vi "Auton - Center Gear.vi"(11 "Auton States":T1=enum."Reset Encoders") -> ()   [LabVIEW 2016]
uses:
  Auton - Center Gear States.ctl
  Robot Values.vi
  Vision Global.vi
panel:
  in  "Turn Setpoint to Mount Peg":dbl=9.0 format="%#_13g"
  in  "Mount Peg Distance SP":dbl=8.0
  out "Current State":T1
  in  "Back Away SP":dbl=-24.0
  in  "Drive Forward SP":dbl=60.0
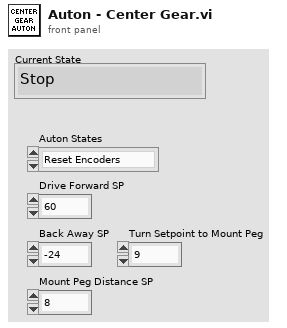
[diagram p1: front panel]
types:
  T1 = typedef "Auton - Center Gear States.ctl" = enum16{"Stop", "Wait For Target", "Reset Encoders", "Drive Forward", "Turn  To Mount Peg", "Reset Encoders Again", "Mount Peg", "Eject Gear", "Back Away"}
  T2 = typedef "Robot Values.ctl" = cluster{"Robot Drive":cluster{"Left Motor Power":dbl, "Right Motor Power":dbl, "Left Encoder Value":dbl, "Right Encoder Value":dbl, "High Gear?":bool, "PTO?":bool}, "Sensors":cluster{"Gyro Angle":u16, "Recalibrate Gyro":bool, "Reset Gyro":bool, "Ultrasonic":dbl}, "Shooter":cluster{"Prep Wheels":bool, "Shoot":bool, "Left Shooter Wheel Speed":dbl, "Wheels Moving":bool, "Shooter Prepped":bool, "Shooter RPS SP":dbl, "Shooting?":bool, "Left Shooter Wheel Power":dbl, "Right Shooter Wheel Power":dbl, "Acquisition Conveyor Power":dbl, "Hopper Beater Bar Power":dbl, "Filtered Left Shooter Speed":dbl, "Acquisition Motor Power":dbl, "Joystick Add":dbl, "D-Pad Add":dbl, "Shooter Use PID?":bool}, "Robot States":cluster{"Drive mode":string, "Alliance":T3, "Position":T4}, "Gear":cluster{"Ejection Active":bool}}
  T3 = typedef "WPI_DriverStationAllianceInfo.ctl" = enum16{"Red", "Blue", "Invalid"}
  T4 = typedef "WPI_DriverStationPositionInfo.ctl" = enum16{"1", "2", "3"}
  T5 = cluster{"Distance (ft)":dbl, "Score":dbl, "Normalized":cluster{"Center":cluster{dbl, dbl}, "Rectangle":cluster{"Numeric":dbl, "Numeric 2":dbl, "Numeric 3":dbl, "Numeric 5":dbl}}, "Pixels":cluster{"Center":cluster{dbl, dbl}, "Rectangle":cluster{"Numeric":dbl, "Numeric 2":dbl, "Numeric 3":dbl, "Numeric 5":dbl}}}
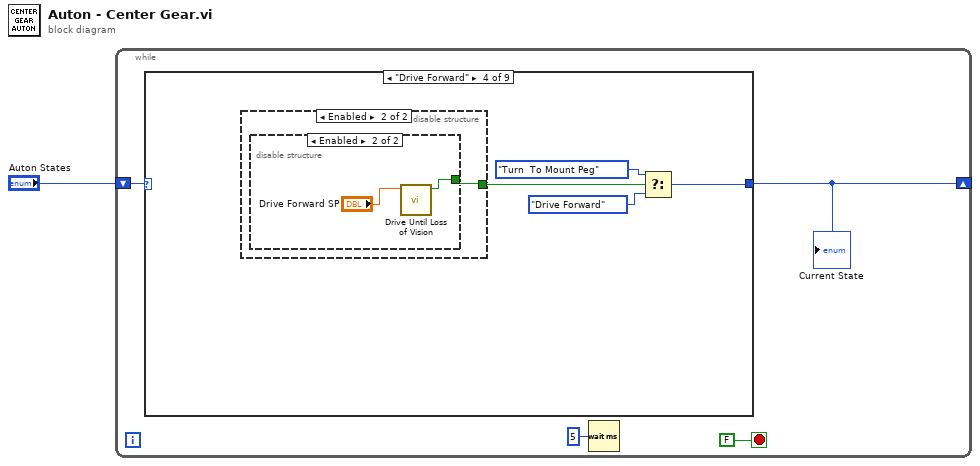
[diagram p0: block diagram]
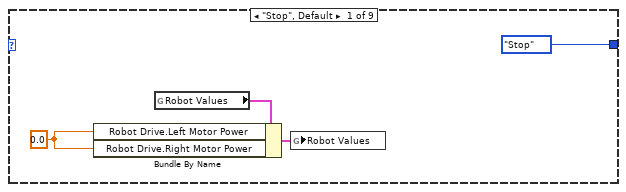
[diagram p2: hidden frame]
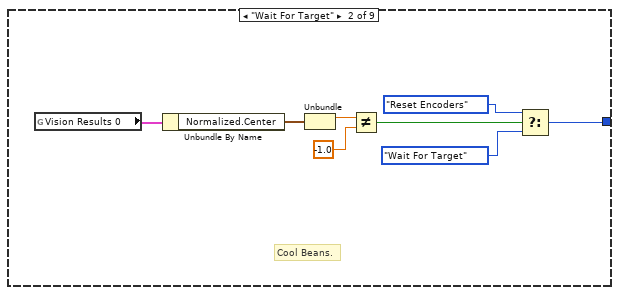
[diagram p3: hidden frame]
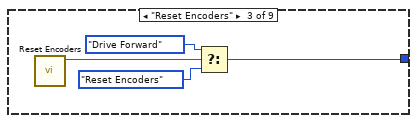
[diagram p4: hidden frame]
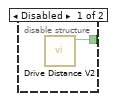
[diagram p5: hidden frame]
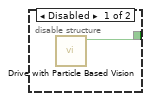
[diagram p6: hidden frame]
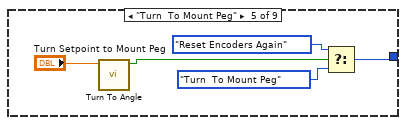
[diagram p7: hidden frame]
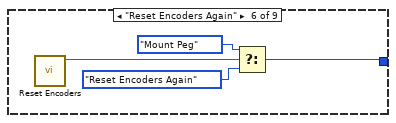
[diagram p8: hidden frame]
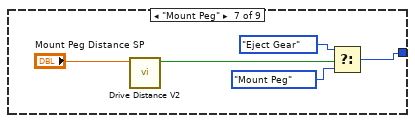
[diagram p9: hidden frame]
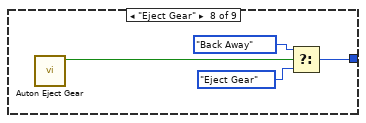
[diagram p10: hidden frame]
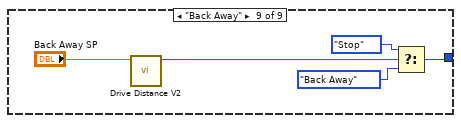
[diagram p11: hidden frame]
diagram:
  n1 = while {
    shift-right: [w4] -> _
    shift-left: "Auton States" -> [w5]
    stop <- FALSE stop-if-true
    n2 = case shown="\"Drive Forward\"" w5 {
      tunnel: [Auton_-_Center_Gear_States."Stop" ("Auton States 2") w17 w19 w23 w34 w37 w42 w47 w52] -> w4
      frame "Stop", Default {
        w6 = 0.0
        n3 = global read "Robot Values.vi" "Robot Values"() -> (w7:T2)
        n4 = Bundle By Name(cluster=w7, "Robot Drive.Left Motor Power"=w6, "Robot Drive.Right Motor Power"=w6) -> (w8:T2)
        n5 = global write "Robot Values.vi" "Robot Values"(w8) -> ()
      }
      frame "Wait For Target" {
        # "Cool Beans."
        n6 = global read "Vision Global.vi" "Vision Results 0"() -> (w14:T5)
        n7 = Unbundle By Name(w14) -> ("Normalized.Center"=w13:cluster{dbl, dbl})
        n8 = Unbundle(w13) -> (w12:dbl)  [unwired: 1 out]
        n9 = Not Equal?(x=w12, y=-1.0) -> (x != y?=w10:bool)
        n10 = Select(t=Auton_-_Center_Gear_States."Reset Encoders" ("Auton States 2"), s=w10, f=Auton_-_Center_Gear_States."Wait For Target") -> (s? t:f=w17:T1)
      }
      frame "Reset Encoders" {
        n11 = call "Reset Encoders.vi"() -> ("Done?"=w18:bool)  [unwired: 11 in]
        n12 = Select(t=Auton_-_Center_Gear_States."Drive Forward" ("Auton States 2"), s=w18, f=Auton_-_Center_Gear_States."Reset Encoders" ("Auton States 2")) -> (s? t:f=w19:T1)
      }
      frame "Drive Forward" {
        n13 = disable-structure shown="Enabled" {
          disable-tunnel: [w27 w28] -> w22
          frame Disabled {
            n14 = call "Drive Distance V2.vi"() -> ("Done?"=w27:bool, "Distance Set Point"=w26:dbl)  [unwired: 10 in]
          }
          frame Enabled {
            n15 = disable-structure shown="Enabled" {
              disable-tunnel: [w29 w31] -> w28
              frame Disabled {
                n16 = call "Drive with Particle Based Vision.vi"() -> ("Done"=w29:bool)  [unwired: 11 in]
              }
              frame Enabled {
                n17 = call "Drive Until Loss of Vision.vi"("Distance Setpoint"="Drive Forward SP") -> ("ready to approach"=w31:bool)  [unwired: 10 in]
              }
            }
          }
        }
        n18 = Select(t=Auton_-_Center_Gear_States."Turn  To Mount Peg" ("Auton States 2"), s=w22, f=Auton_-_Center_Gear_States."Drive Forward" ("Auton States 2")) -> (s? t:f=w23:T1)
      }
      frame "Turn  To Mount Peg" {
        n19 = call "Turn To Angle.vi"("Setpoint"="Turn Setpoint to Mount Peg") -> ("Done?"=w33:bool)  [unwired: 10 in]
        n20 = Select(t=Auton_-_Center_Gear_States."Reset Encoders Again" ("Auton States 2"), s=w33, f=Auton_-_Center_Gear_States."Turn  To Mount Peg" ("Auton States 2")) -> (s? t:f=w34:T1)
      }
      frame "Reset Encoders Again" {
        n21 = call "Reset Encoders.vi"() -> ("Done?"=w38:bool)  [unwired: 11 in]
        n22 = Select(t=Auton_-_Center_Gear_States."Mount Peg" ("Auton States 2"), s=w38, f=Auton_-_Center_Gear_States."Reset Encoders Again" ("Auton States 2")) -> (s? t:f=w37:T1)
      }
      frame "Mount Peg" {
        n23 = call "Drive Distance V2.vi"("Distance Set Point"="Mount Peg Distance SP") -> ("Done?"=w41:bool)  [unwired: 10 in]
        n24 = Select(t=Auton_-_Center_Gear_States."Eject Gear" ("Auton States 2"), s=w41, f=Auton_-_Center_Gear_States."Mount Peg" ("Auton States 2")) -> (s? t:f=w42:T1)
      }
      frame "Eject Gear" {
        n25 = call "Auton Eject Gear.vi"() -> ("Done?"=w46:bool)  [unwired: 11 in]
        n26 = Select(t=Auton_-_Center_Gear_States."Back Away" ("Auton States 2"), s=w46, f=Auton_-_Center_Gear_States."Eject Gear" ("Auton States 2")) -> (s? t:f=w47:T1)
      }
      frame "Back Away" {
        n27 = call "Drive Distance V2.vi"("Distance Set Point"="Back Away SP") -> ("Done?"=w51:bool)  [unwired: 10 in]
        n28 = Select(t=Auton_-_Center_Gear_States."Stop" ("Auton States 2"), s=w51, f=Auton_-_Center_Gear_States."Back Away" ("Auton States 2")) -> (s? t:f=w52:T1)
      }
    }
    "Current State" <- w4
    n29 = Wait (ms)(milliseconds to wait=u32 5) -> ()  [unwired: 1 out]
  }
